vi "clLabview_writeToFile.vi"(8 "filename (use dialog)":path, 11 "vi_lib.lvlib:clLabview.lvclass":refnum<class "clLabview.lvclass">) -> (0 "no Error":bool, 3 "vi_lib.lvlib:clLabview.lvclass 2":refnum<class "clLabview.lvclass">)   [LabVIEW 2011, in "vi_lib.lvlib" / "clLabview.lvclass"]
uses:
  clLabview.lvclass
  clLabview.lvclass/clLabview.ctl
  clFileReader/clFileReader.lvclass
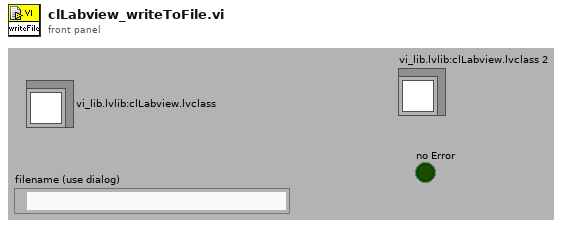
[diagram p1: front panel]
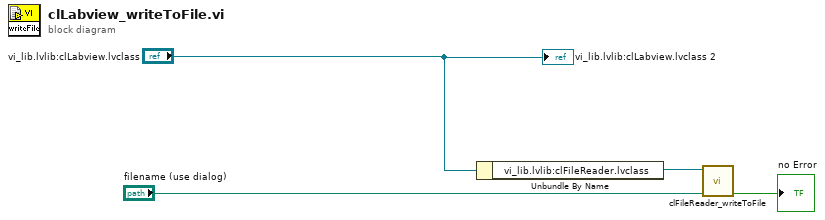
[diagram p0: block diagram]
diagram:
  n1 = Unbundle By Name("vi_lib.lvlib:clLabview.lvclass") -> ("vi_lib.lvlib:clFileReader.lvclass"=w3:refnum<class "clFileReader.lvclass">)
  n2 = call "clFileReader_writeToFile.vi"("filename (use dialog)"="filename (use dialog)", "clFileReader.lvclass IN"=w3) -> ("no Error"=→"no Error":bool)  [unwired: 9 out]
  "vi_lib.lvlib:clLabview.lvclass 2" <- "vi_lib.lvlib:clLabview.lvclass"
